vi "Problem1.10.vi"() -> ()   [LabVIEW 2019]
uses:
  <vilib>/Analysis/baseanly.llb/Mean (DBL).vi
  <vilib>/Analysis/NI_AALBase.lvlib
panel:
  out "Random Number Array":dbl[](array[numeric])
  out "Histogram":dynamicdata(graph)
  out "Uniform Deviate Array":dbl[](array[numeric])
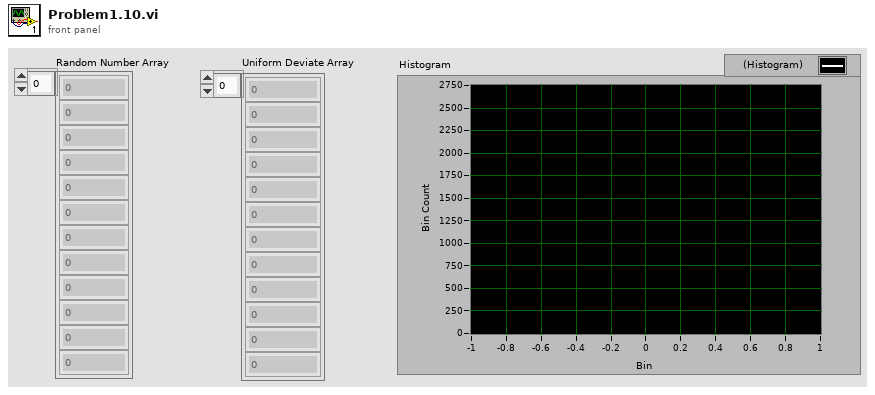
[diagram p1: front panel]
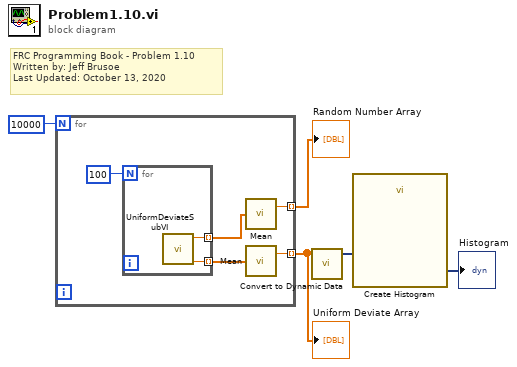
[diagram p0: block diagram]
diagram:
  # "FRC Programming Book - Problem 1.10\nWritten by: Jeff Brusoe\nLast Updated: October 13, 2020"
  n1 = for {
    N: 10000 -> [_]
    tunnel: [w8] -> w2 mode=indexing
    tunnel: [w6] -> w1 mode=indexing
    n2 = for {
      N: 100 -> [_]
      tunnel: [w12] -> w9 mode=indexing
      tunnel: [w11] -> w7 mode=indexing
      n3 = call "UniformDeviateSubVI.vi"() -> ("Uniform Deviate"=w12:dbl, "Initial Random Number"=w11:dbl)  [unwired: 10 in]
    }
    n4 = call-poly <vilib>:"Mean.vi"("X"=w7) -> ("mean"=w6:dbl)  [unwired: 1 out]
    n5 = call-poly <vilib>:"Mean.vi"("X"=w9) -> ("mean"=w8:dbl)  [unwired: 1 out]
  }
  "Uniform Deviate Array" <- w2
  "Random Number Array" <- w1
  n6 = call "Convert to Dynamic Data"("Array"=w2) -> ("Dynamic Data Type"=w4:dynamicdata)  [unwired: 3 in]
  n7 = call "Create Histogram"("Signal"=w4) -> ("Histogram"=→"Histogram":dynamicdata)  [unwired: 9 in, 1 out]
